vi "folderPathFromPath.vi"(11 "File Path Control":path) -> (3 "stripped path":path)   [LabVIEW 2020]
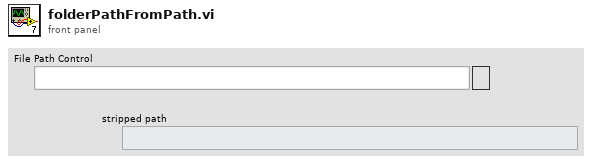
[diagram p1: front panel]
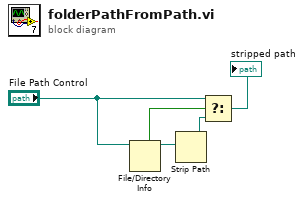
[diagram p0: block diagram]
diagram:
  n1 = File/Directory Info(path="File Path Control") -> (path out=w2:path, directory=w5:bool)  [unwired: 1 in, 5 out]
  n2 = Strip Path(path=w2) -> (stripped path=w1:path)  [unwired: 1 out]
  n3 = Select(t="File Path Control", s=w5, f=w1) -> (s? t:f=→"stripped path":path)
